vi "to string.vi"(8 "error in":errorcluster, 11 "asynchronous execution module configuration In":refnum<class "asynchronous execution module configuration.lvclass">) -> (0 "error out":errorcluster, 1 "data":string, 2 "version":string, 3 "asynchronous execution module configuration Out":refnum<class "asynchronous execution module configuration.lvclass">)   [LabVIEW 2013, in "asynchronous execution module configuration.lvclass"]
doc: "Provides an interface for saving a component configuration to a file or other serialized data source. It is recommended that all children of this class store data in two sets--data required for its own initialization, and any data required for parent initialization--and that each implementation uses the <b>Call Parent Method</b> primitive to serialize parent information."
uses:
  asynchronous execution module configuration.lvclass
  <vilib>/NI/Tag Bus Module Framework/module configuration/TBM module configuration.lvclass
  asynchronous execution module configuration.lvclass/asynchronous execution module configuration.ctl
  current version.vi
  <vilib>/NI/Tag Bus Module Framework/root configuration/TBM configuration.lvclass
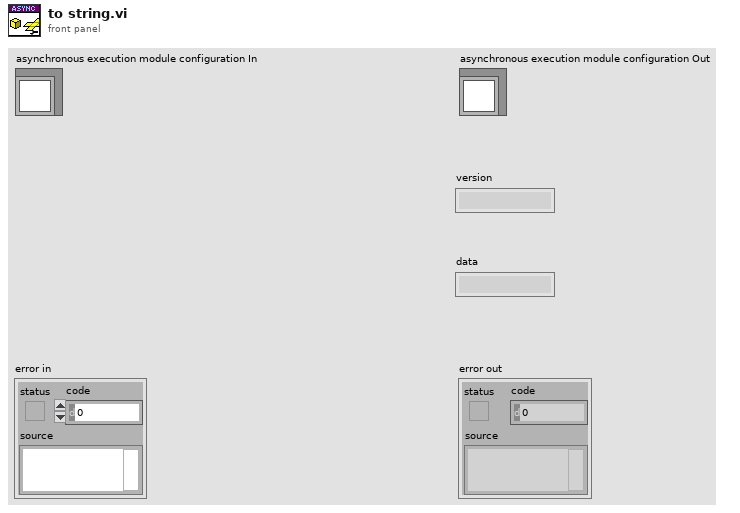
[diagram p1: front panel]
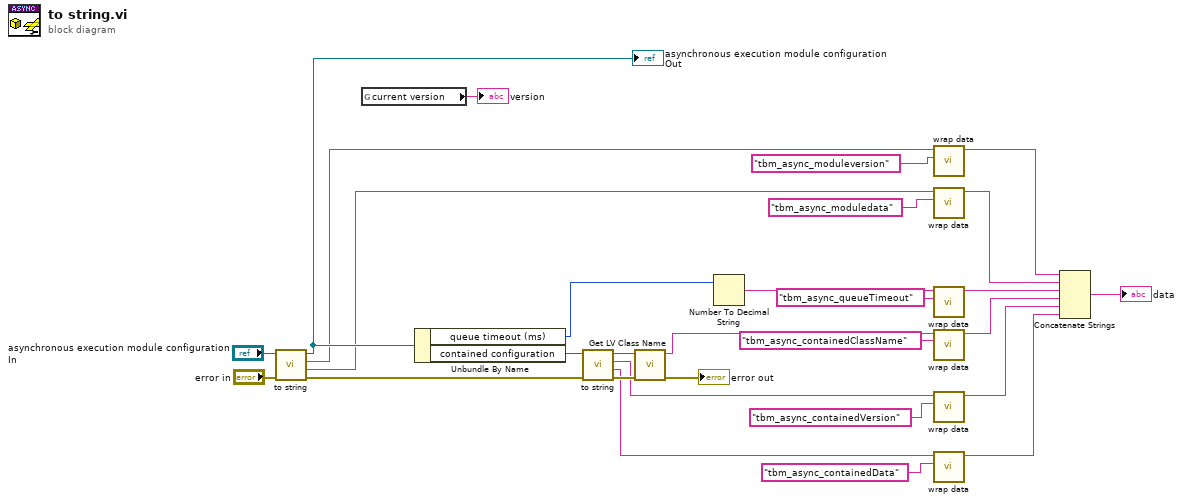
[diagram p0: block diagram]
diagram:
  n1 = call-parent "to string.vi"("error in"="error in", "module configuration in"="asynchronous execution module configuration In") -> ("error out"=w24:errorcluster, "data"=w16:string, "version"=w17:string, "module configuration out"=w26:refnum<class "asynchronous execution module configuration.lvclass">)  [unwired: 6 in]
  "asynchronous execution module configuration Out" <- w26
  n2 = global read "current version.vi" "current version"() -> (→"version":string)
  n3 = Unbundle By Name(w26) -> ("queue timeout (ms)"=w2:i32, "contained configuration"=w25:refnum<class "TBM module configuration.lvclass">)
  n4 = call-dynamic "to string.vi"("error in"=w24, "module configuration in"=w25) -> ("error out"=w22:errorcluster, "data"=w11:string, "version"=w12:string, "module configuration out"=w23:refnum<class "TBM module configuration.lvclass">)  [unwired: 6 in]
  n5 = call <vilib>:"Get LV Class Name.vi"("error in (no error)"=w22, "object"=w23) -> ("error out"=→"error out":errorcluster, "class name"=w13:string)  [unwired: 8 in]
  n6 = Number To Decimal String(number=w2) -> (decimal integer string=w1:string)  [unwired: 1 in]
  n7 = call <vilib>:"wrap data.vi"("identifier"="tbm_async_moduleversion" ("additional identifier"), "data to wrap"=w17) -> ("wrapped data"=w9:string)  [unwired: 9 in]
  n8 = call <vilib>:"wrap data.vi"("identifier"="tbm_async_moduledata" ("additional identifier"), "data to wrap"=w16) -> ("wrapped data"=w8:string)  [unwired: 9 in]
  n9 = call <vilib>:"wrap data.vi"("identifier"="tbm_async_queueTimeout" ("additional identifier"), "data to wrap"=w1) -> ("wrapped data"=w7:string)  [unwired: 9 in]
  n10 = call <vilib>:"wrap data.vi"("identifier"="tbm_async_containedClassName" ("additional identifier"), "data to wrap"=w13) -> ("wrapped data"=w6:string)  [unwired: 9 in]
  n11 = call <vilib>:"wrap data.vi"("identifier"="tbm_async_containedVersion" ("additional identifier"), "data to wrap"=w12) -> ("wrapped data"=w5:string)  [unwired: 9 in]
  n12 = call <vilib>:"wrap data.vi"("identifier"="tbm_async_containedData" ("additional identifier"), "data to wrap"=w11) -> ("wrapped data"=w4:string)  [unwired: 9 in]
  n13 = Concatenate Strings(w9, w8, w7, w6, w5, w4) -> (→"data":string)
